vi "TEST - Object Cluster Equivalence.vi"(8 "error in (no error)":errorcluster) -> (0 "error out":errorcluster, 2 "pass":bool)   [LabVIEW 2020, in "test_openg_array.lvlib"]
uses:
  test_openg_array.lvlib
  LVOOP Data/Subclass Data/Subclass Data.lvclass
  source/library/openg_variant.lvlib
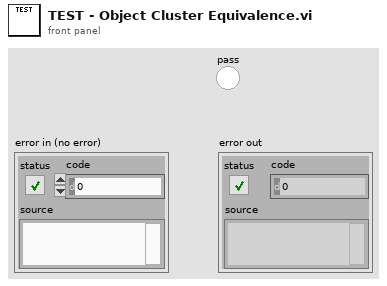
[diagram p1: front panel]
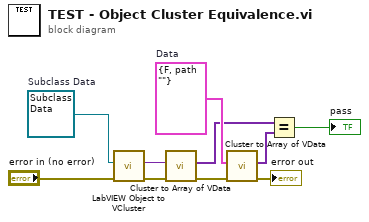
[diagram p0: block diagram]
diagram:
  w10 = cluster{"Boolean":bool, "Path":path} {"Boolean"=FALSE, "Path"=path ""}  # Data
  w9 = refnum<class "Subclass Data.lvclass"> refnum  # Subclass Data
  n1 = call "LabVIEW Object to VCluster.vi"("error in (no error)"="error in (no error)", "LabVIEW Object"=w9) -> ("error out"=w4:errorcluster, "VCluster"=w5:variant)  [unwired: 8 in]
  n2 = call "Cluster to Array of VData.vi"("error in (no error)"=w4, "Cluster"=w5) -> ("error out"=w2:errorcluster, "Array of VData"=w7:variant[])  [unwired: 8 in]
  n3 = call "Cluster to Array of VData.vi"("error in (no error)"=w2, "Cluster"=w10) -> ("error out"=→"error out":errorcluster, "Array of VData"=w8:variant[])  [unwired: 8 in]
  n4 = Equal?(x=w7, y=w8) -> (x = y?=→"pass":bool)
